vi "3.vi"(1 "停止":bool, 2 "温度单位":bool) -> (0 "温度计":dbl(slide) scale=0.0..100.0, 3 "结果字符串":string)   [LabVIEW 2017]
panel:
  # "℃"
  # "℉"
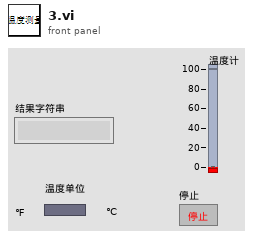
[diagram p1: front panel]
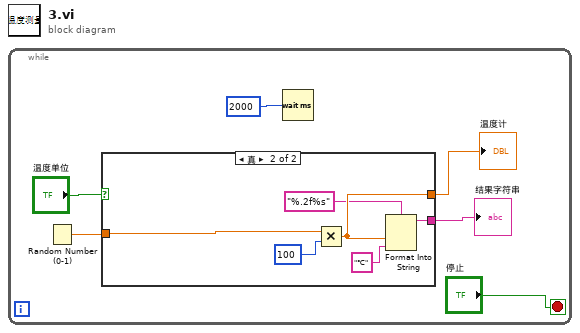
[diagram p0: block diagram]
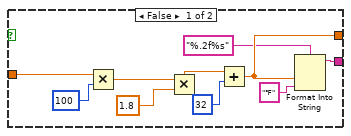
[diagram p2: hidden frame]
diagram:
  n1 = while {
    stop <- "停止" stop-if-true
    n2 = Random Number (0-1)() -> (number: 0 to 1=w3:dbl)
    n3 = case shown="真" "温度单位" {
      tunnel: [w11 w20] -> w6
      tunnel: [w8 w19] -> w4
      tunnel: w3 -> [w7 w17]
      frame False {
        n4 = Multiply(x=w7, y=100) -> (x*y=w15:dbl)
        n5 = Multiply(x=w15, y=1.8) -> (x*y=w13:dbl)
        n6 = Add(x=w13, y=32) -> (x+y=w11:dbl)
        n7 = Format Into String(format string="%.2f%s", w11, "℉") -> (resulting string=w8:string)  [unwired: 2 in, 1 out]
      }
      frame True {
        n8 = Multiply(x=w17, y=100) -> (x*y=w20:dbl)
        n9 = Format Into String(format string="%.2f%s", w20, "℃") -> (resulting string=w19:string)  [unwired: 2 in, 1 out]
      }
    }
    "温度计" <- w6
    "结果字符串" <- w4
    n10 = Wait (ms)(milliseconds to wait=2000) -> ()  [unwired: 1 out]
  }
